vi "Subvi.vi"() -> ()   [LabVIEW 2017]
panel:
  in  "legth (rest)":i32=32
  in  "offset (0)":i32=69
  in  "string":string
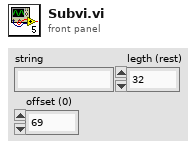
[diagram p1: front panel]
types:
  T1 = enum16{"Char", "DBL", "SGL", "I64", "I32", "I16", "I8", "U64", "U32", "U16", "U8"}
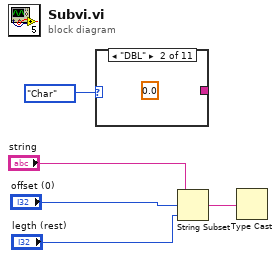
[diagram p0: block diagram]
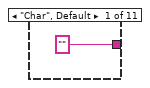
[diagram p2: hidden frame]
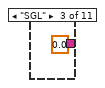
[diagram p3: hidden frame]
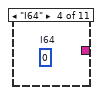
[diagram p4: hidden frame]
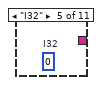
[diagram p5: hidden frame]
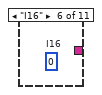
[diagram p6: hidden frame]
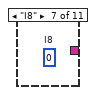
[diagram p7: hidden frame]
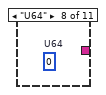
[diagram p8: hidden frame]
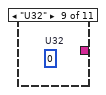
[diagram p9: hidden frame]
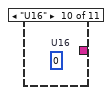
[diagram p10: hidden frame]
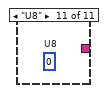
[diagram p11: hidden frame]
diagram:
  n1 = case shown="\"DBL\"" T1."Char" {
    tunnel: ["" _ _ _ _ _ _ _ _ _ _] -> _
    frame "Char", Default {
    }
    frame "DBL" {
      (unwired) 0.0
    }
    frame "SGL" {
      (unwired) sgl 0.0
    }
    frame "I64" {
      (unwired) i64 0  # I64
    }
    frame "I32" {
      (unwired) 0  # I32
    }
    frame "I16" {
      (unwired) i16 0  # I16
    }
    frame "I8" {
      (unwired) i8 0  # I8
    }
    frame "U64" {
      (unwired) u64 0  # U64
    }
    frame "U32" {
      (unwired) u32 0  # U32
    }
    frame "U16" {
      (unwired) u16 0  # U16
    }
    frame "U8" {
      (unwired) u8 0  # U8
    }
  }
  n2 = String Subset(string="string", offset (0)="offset (0)", length (rest)="legth (rest)") -> (substring=w3:string)
  n3 = Type Cast(x=w3) -> ()  [unwired: 1 in, 1 out]
